vi "Select Function.vi"() -> ()   [LabVIEW 2020]
panel:
  out "Result":dbl
  in  "Random Number?":bool
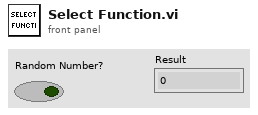
[diagram p1: front panel]
types:
  T1 = enum16{"open", "replace", "create", "open or create", "replace or create", "replace or create with confirmation"}
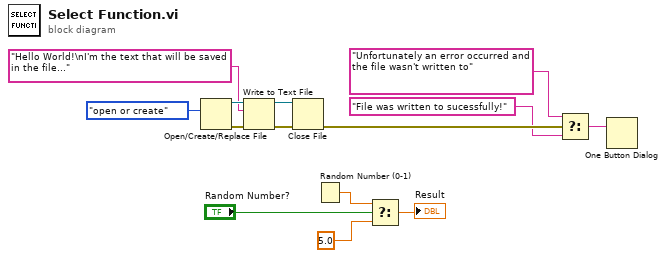
[diagram p0: block diagram]
diagram:
  n1 = Open/Create/Replace File(operation (0:open)=T1."open or create") -> (refnum out=w10:refnum<file>, error out=w9:errorcluster)  [unwired: 5 in, 1 out]
  n2 = Write to Text File(file (use dialog)=w10, text="Hello World!\nI'm the text that will be saved in the file...", error in=w9) -> (refnum out=w8:refnum<file>, error out=w7:errorcluster)  [unwired: 1 in, 1 out]
  n3 = Close File(refnum=w8, error in=w7) -> (error out=w4:errorcluster)  [unwired: 1 out]
  n4 = Random Number (0-1)() -> (number: 0 to 1=w13:dbl)
  n5 = Select(t=w13, s="Random Number?", f=5.0 ("t")) -> (s? t:f=→"Result":dbl)
  n6 = Select(t="Unfortunately an error occurred and the file wasn't written to", s=w4, f="File was written to sucessfully!") -> (s? t:f=w3:string)
  n7 = One Button Dialog(message=w3) -> ()  [unwired: 1 in, 1 out]
